vi "UART Set Baud Rate.vi"(8 "Error In":errorcluster, 9 "Baud Rate (9600)":u32=9600, 10 "UART Channel (0)":u8, 11 "LINX Resource":T1) -> (0 "Error Out":errorcluster, 3 "LINX Resource":T1)   [LabVIEW 2013, in "LVH-LINX.lvlib"]
doc: "Set the buad rate of the specified UART channel."
uses:
  <vilib>/LabVIEW Hacker/LINX/LVH-LINX.lvlib
  <vilib>/LabVIEW Hacker/LINX/Private/Type Defs/LINX Ref.ctl
  <vilib>/LabVIEW Hacker/LINX/Private/Type Defs/Platform.ctl
  <vilib>/LabVIEW Hacker/LINX/Private/Type Defs/Interface.ctl
  <vilib>/LabVIEW Hacker/LINX/Private/Device/Type Defs/LINX Device Config.ctl
  <vilib>/LabVIEW Hacker/LINX/Private/Device/Type Defs/TCP Config.ctl
  <vilib>/LabVIEW Hacker/LINX/Private/Type Defs/Device Family.ctl
  <vilib>/LabVIEW Hacker/LINX/Private/Type Defs/Peripheral.ctl
  <vilib>/LabVIEW Hacker/LINX/Private/Type Defs/Channel FGV States.ctl
  <vilib>/Instr/_visa.llb/VISA Configure Serial Port (Instr).vi
  <vilib>/LabVIEW Hacker/LINX/Private/myRIO/myRIO.lvlib
  <vilib>/LabVIEW Hacker/LINX/Private/Device/Device.lvlib
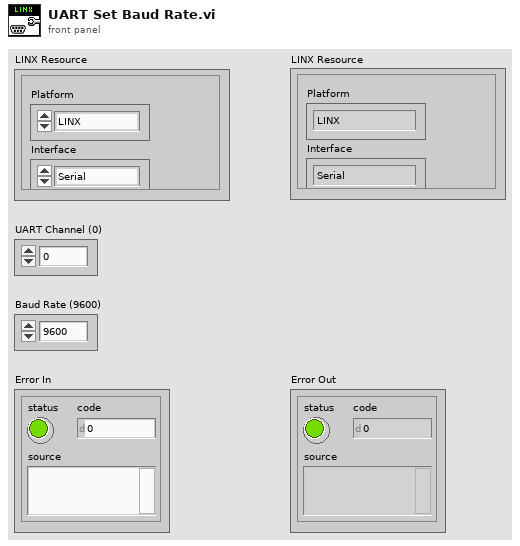
[diagram p1: front panel]
types:
  T1 = typedef "LVH-LINX.lvlib/LINX Ref.ctl" = cluster{"Platform":T2, "Interface":T3, "LINX Device Config":T4}
  T2 = typedef "LVH-LINX.lvlib/Platform.ctl" = enum16{"LINX", "myRIO"}
  T3 = typedef "LVH-LINX.lvlib/Interface.ctl" = enum16{"Serial", "TCP"}
  T4 = typedef "LVH-LINX.lvlib/Device.lvlib/LINX Device Config.ctl" = cluster{"Interface":T3, "COM Port":refnum<visa-resource-name>, "TCP Configuration":T5, "Device Family":T6, "Device ID":u8, "Device Name":string, "TCP Ref":refnum<k5>}
  T5 = typedef "LVH-LINX.lvlib/Device.lvlib/TCP Config.ctl" = cluster{"IP Address":string, "Port":u16}
  T6 = typedef "LVH-LINX.lvlib/Device Family.ctl" = enum8{"National Instruments", "Digilent", "Arduino"}
  T7 = typedef "LVH-LINX.lvlib/Peripheral.ctl" = enum8{"DI", "DO", "AI", "AO", "PWM", "QE", "UART", "I2C", "SPI", "CAN"}
  T8 = typedef "LVH-LINX.lvlib/Channel FGV States.ctl" = enum16{"Initialize", "Get", "Set"}
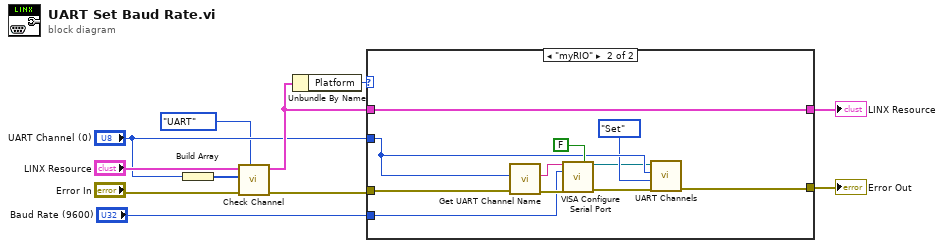
[diagram p0: block diagram]
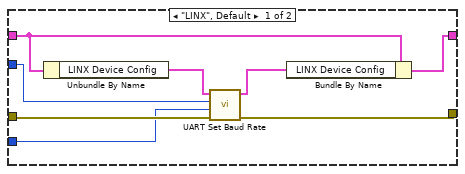
[diagram p2: hidden frame]
diagram:
  n1 = Build Array("UART Channel (0)") -> (w4:u8[])
  n2 = call <vilib>:"Check Channel.vi"("Peripheral"=Peripheral."UART", "Error In"="Error In", "Channels"=w4, "LINX Resource"="LINX Resource") -> ("Error Out"=w5:errorcluster, "LINX Resource"=w6:T1)  [unwired: 5 in, 1 out]
  n3 = Unbundle By Name(w6) -> ("Platform"=w11:T2)
  n4 = case shown="\"myRIO\"" w11 {
    tunnel: w5 -> [w16 w23]
    tunnel: w6 -> [w19 w30]
    tunnel: [w17 w21] -> w10
    tunnel: [w18 w30] -> w9
    tunnel: "UART Channel (0)" -> [w13 w25]
    tunnel: "Baud Rate (9600)" -> [w12 w27]
    frame "LINX", Default {
      n5 = Unbundle By Name(w19) -> ("LINX Device Config"=w14:T4)
      n6 = call <vilib>:"UART Set Baud Rate.vi"("Error In"=w16, "Baud Rate (9600)"=w12, "UART Channel"=w13, "LINX Device Config"=w14) -> ("Error Out"=w17:errorcluster, "LINX Device Config"=w15:T4)  [unwired: 6 in]
      n7 = Bundle By Name(cluster=w19, "LINX Device Config"=w15) -> (w18:T1)
    }
    frame "myRIO" {
      n8 = call <vilib>:"Get UART Channel Name.vi"("Error In"=w23, "UART Channel"=w25) -> ("Error Out"=w28:errorcluster, "UART Channel"=w26:string)  [unwired: 8 in]
      n9 = call-poly "VISA Configure Serial Port"("VISA resource name"=w26, "Enable Termination\nChar (T)"=FALSE ("Enable Termination\nChar (T)"), "baud rate (9600)"=w27, "error in (no error)"=w28) -> ("VISA resource name out"=w20:refnum<visa-resource-name>, "error out"=w22:errorcluster)  [unwired: 10 in]
      n10 = call <vilib>:"UART Channels.vi"("Error In"=w22, "Channel State"=Channel_FGV_States."Set", "Channel Number"=w25, "UART Channel"=w20) -> ("Error Out"=w21:errorcluster)  [unwired: 6 in, 1 out]
    }
  }
  "Error Out" <- w10
  "LINX Resource" <- w9
